vi "Reference pressure module - Get ident.vi"() -> ()   [LabVIEW 2020]
uses:
  Arduino/ctls_and_globals/Arduino tx msg cluster.ctl
panel:
  out "Ident":string
  out "Scan comment":string
  in  "Port":refnum<visa-resource-name>
  in  "Address":u8=1
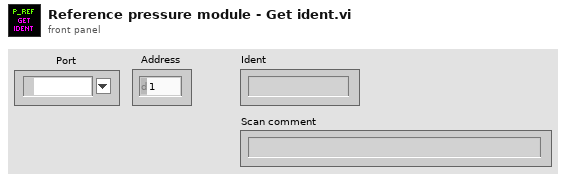
[diagram p1: front panel]
types:
  T1 = typedef "Arduino tx msg cluster.ctl" = cluster{"dest":u8, "A/D/C/I":string, "R/W":string, "chan":u8, "val (float)":sgl}
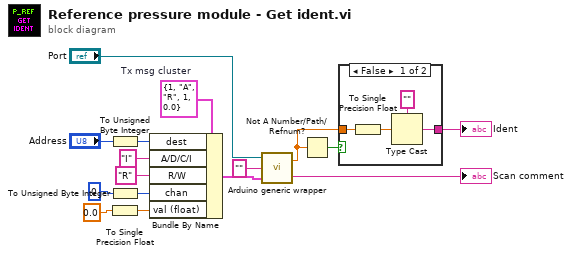
[diagram p0: block diagram]
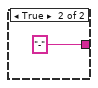
[diagram p2: hidden frame]
diagram:
  w14 = T1 {"dest"=1, "A/D/C/I"="A", "R/W"="R", "chan"=1, "val (float)"=0.0}  # Tx msg cluster
  n1 = To Unsigned Byte Integer(number="Address") -> (unsigned 8bit integer=w12:u8)
  n2 = To Unsigned Byte Integer(number=u8 0) -> (unsigned 8bit integer=w13:u8)
  n3 = To Single Precision Float(number=0.0) -> (single precision float=w10:sgl)
  n4 = Bundle By Name(cluster=w14, "dest"=w12, "A/D/C/I"="I" ("A/D"), "R/W"="R", "chan"=w13, "val (float)"=w10) -> (w11:T1)
  n5 = call "Arduino generic wrapper.vi"("Tx msg cluster"=w11, "Channel Name"="", "Port name"="Port") -> ("Scan comment"=→"Scan comment":string, "Output"=w2:dbl)
  n6 = Not A Number/Path/Refnum?(number/path/refnum=w2) -> (NaN/Path/Refnum?=w3:bool)
  n7 = case shown="False" w3 {
    tunnel: w2 -> [w18 _]
    tunnel: [w19 "-"] -> w1
    frame False {
      n8 = To Single Precision Float(number=w18) -> (single precision float=w17:sgl)
      n9 = Type Cast(type="", x=w17) -> (*(type *) &x=w19:string)
    }
    frame True {
    }
  }
  "Ident" <- w1
